vi "Six 8-bit Port Digital Input.vi"(2 "Six 8-bit DI Ports":T1={"8-bit DI Port 0"="Chassis1/Mod4/DI7:0", "8-bit DI Port 1"="Chassis1/Mod4/DI7:0", "8-bit DI Port 2"="Chassis1/Mod4/DI7:0", "8-bit DI Port 3"="Chassis1/Mod4/DI7:0", "8-bit DI Port 4"="Chassis1/Mod4/DI7:0", "8-bit DI Port 5"="Chassis1/Mod4/DI7:0"}) -> (7 "Packet":u64)   [LabVIEW 2009]
uses:
  <vilib>/eio/EIONode/EIONode.xnode
  <vilib>/rvi/eio/nirviEIOImplementation/nirviEIOImplementation.xnode
  <vilib>/rvi/eio/common/nirviEmuTemplateMethod_noerrors.vi
  <vilib>/rvi/eio/common/nirviEmuClasses.ctl
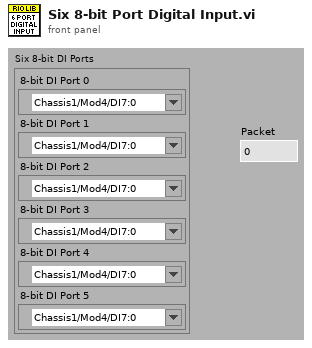
[diagram p1: front panel]
types:
  T1 = cluster{"8-bit DI Port 0":refnum<k21>, "8-bit DI Port 1":refnum<k21>, "8-bit DI Port 2":refnum<k21>, "8-bit DI Port 3":refnum<k21>, "8-bit DI Port 4":refnum<k21>, "8-bit DI Port 5":refnum<k21>}
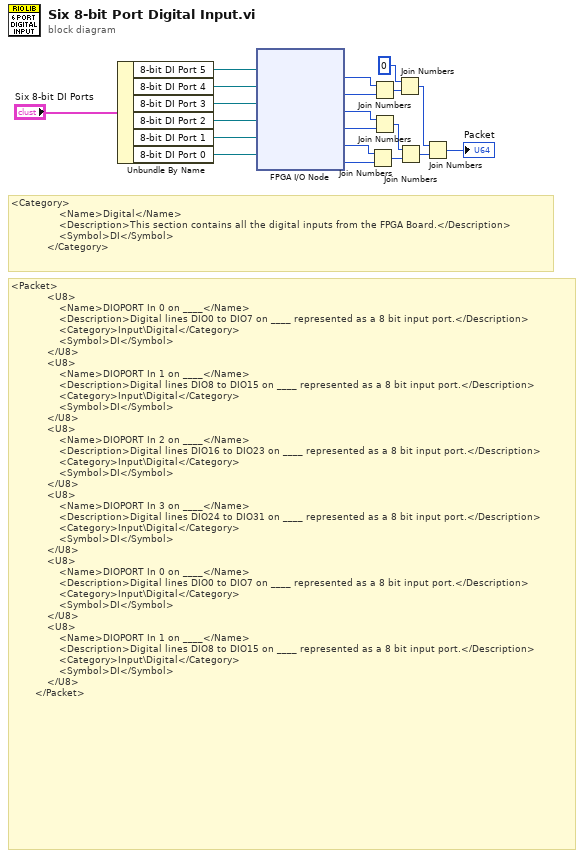
[diagram p0: block diagram]
diagram:
  # "<Packet>\n            <U8>\n                <Name>DIOPORT In 0 on ____</Name>\n                <Description>Digital lines DIO0 to DIO7 on ____ represented as a 8 bit input port.</Description>\n                <Category>Input\\Digital</Category>\n                <Symbol>DI</Symbol>\n            </U8>\n            <U8>\n                <Name>DIOPORT In 1 on ____</Name>\n                <Description>Digital lines DIO8 to DIO15 on ____ represented as a 8 bit input port.</Description>\n                <Category>Input\\Digital</Category>\n                <Symbol>DI</Symbol>\n            </U8>\n            <U8>\n                <Name>DIOPORT In 2 on ____</Name>\n                <Description>Digital lines DIO16 to DIO23 on ____ represented as a 8 bit input port.</Description>\n                <Category>Input\\Digital</Category>\n                <Symbol>DI</Symbol>\n            </U8>\n            <U8>\n                <Name>DIOPORT In 3 on ____</Name>\n                <Description>Digital lines DIO24 to DIO31 on ____ represented as a 8 bit input port.</Description>\n                <Category>Input\\Digital</Category>\n                <Symbol>DI</Symbol>\n            </U8>\n            <U8>\n                <Name>DIOPORT In 0 on ____</Name>\n                <Description>Digital lines DIO0 to DIO7 on ____ represented as a 8 bit input port.</Description>\n                <Category>Input\\Digital</Category>\n                <Symbol>DI</Symbol>\n            </U8>\n            <U8>\n                <Name>DIOPORT In 1 on ____</Name>\n                <Description>Digital lines DIO8 to DIO15 on ____ represented as a 8 bit input port.</Description>\n                <Category>Input\\Digital</Category>\n                <Symbol>DI</Symbol>\n            </U8>\n        </Packet>"
  # "<Category>\n                <Name>Digital</Name>\n                <Description>This section contains all the digital inputs from the FPGA Board.</Description>\n                <Symbol>DI</Symbol>\n            </Category>"
  n1 = Unbundle By Name("Six 8-bit DI Ports") -> ("8-bit DI Port 5"=w2:refnum<k21>, "8-bit DI Port 4"=w7:refnum<k21>, "8-bit DI Port 3"=w9:refnum<k21>, "8-bit DI Port 2"=w13:refnum<k21>, "8-bit DI Port 1"=w15:refnum<k21>, "8-bit DI Port 0"=w16:refnum<k21>)
  n2 = xnode "FPGA I/O Node"("FPGA I/O In"=w2, "FPGA I/O In"=w7, "FPGA I/O In"=w9, "FPGA I/O In"=w13, "FPGA I/O In"=w15, "FPGA I/O In"=w16) -> ("I/O Item"=w1:u8, "I/O Item"=w4:u8, "I/O Item"=w8:u8, "I/O Item"=w11:u8, "I/O Item"=w14:u8, "I/O Item"=w19:u8)  [unwired: 6 out]
  n3 = Join Numbers(hi=w14, lo=w19) -> ((hi.lo)=w12:u16)
  n4 = Join Numbers(hi=w1, lo=w4) -> ((hi.lo)=w6:u16)
  n5 = Join Numbers(hi=w8, lo=w11) -> ((hi.lo)=w10:u16)
  n6 = Join Numbers(hi=u8 0, lo=w6) -> ((hi.lo)=w5:u32)
  n7 = Join Numbers(hi=w10, lo=w12) -> ((hi.lo)=w20:u32)
  n8 = Join Numbers(hi=w5, lo=w20) -> ((hi.lo)=→"Packet":u64)
